vi "Bilan.vi"(1 "Argent ventes":dbl, 2 "Dettes":dbl) -> (0 "Bilan":dbl)   [LabVIEW 2024]
uses:
  charge_salairial.vi
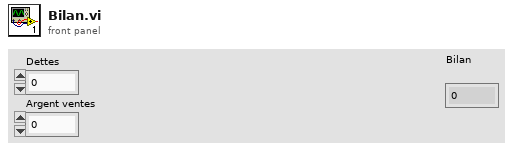
[diagram p1: front panel]
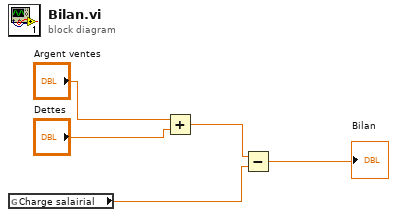
[diagram p0: block diagram]
diagram:
  n1 = global read "charge_salairial.vi" "Charge salairial"() -> (w3:dbl)
  n2 = Add(x="Argent ventes", y="Dettes") -> (x+y=w2:dbl)
  n3 = Subtract(x=w2, y=w3) -> (x-y=→"Bilan":dbl)
